vi "Shooter Published Globals.vi"() -> ()   [LabVIEW 2020]
doc: "This is used primarily to publish values that other subsystems or user code may want to read periodically. It may also contain some settings such as debug switches or implementation selections that are independent of the operating mode of the subsystem."
uses:
  Shooter Setpoints.ctl
  Shooter Operations.ctl
  <vilib>/Rock Robotics/WPI/Framework/Command Status Info.ctl
  <vilib>/Rock Robotics/WPI/Framework/Completion Status.ctl
  <vilib>/Rock Robotics/WPI/Framework/Completion Notifier.ctl
panel:
  in  "Current Command":T6
  # "Tip: The global is a good way publish state or\ninformational/debugging values.\nIt is not  advised that you put setpoint values here."
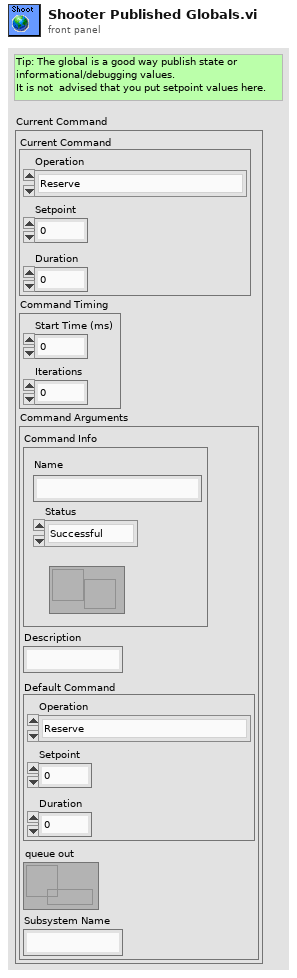
[diagram p1: front panel]
types:
  T1 = typedef "Shooter Setpoints.ctl" = cluster{"Operation":T2, "Setpoint":dbl, "Duration":dbl}
  T2 = typedef "Shooter Operations.ctl" = enum16{"Reserve", "Read Current", "Immediate", "with Duration", "Stop"}
  T3 = typedef "Command Status Info.ctl" = cluster{"Name":string, "Status":T4, "notifier out":T5}
  T4 = typedef "Completion Status.ctl" = enum16{"Successful", "Aborted", "Incomplete"}
  T5 = typedef "Completion Notifier.ctl" = refnum<notifier>
  T6 = cluster{"Current Command":T1, "Command Timing":cluster{"Start Time (ms)":u32, "Iterations":i32}, "Command Arguments":cluster{"Command Info":T3, "Description":string, "Default Command":T1, "queue out":refnum<queue>, "Subsystem Name":string}}
diagram:
